vi "Detect Network Devices.vi"(4 "Remote Timeout":u32=300000 caption="Remote Timeout (300,000 ms)", 6 "Network Adapters":bool caption="Network Adapters (F)", 7 "Local Subnet Only":bool caption="Local Subnet Only (F)", 8 "Error in":errorcluster, 11 "Session in (localhost)":refnum<k21>="localhost") -> (0 "Error out":errorcluster, 1 "Devices Skipped":T1[](array[typedef]) {"Network Adapter Settings"."IP Address Request Mode" items=["Static"=1, "DHCP/Link Local"=2, "Link-Local Only"=4, "DHCP Only"=8]; "Network Adapter Settings"."Adapter Type" items=["Disabled"=1, "TCP/IP Ethernet"=2, "Deterministic"=4, "EtherCAT"=8, "TCP/IP WLAN Connect"=32, "TCP/IP WLAN Create"=64]; "Network Adapter Settings"."Adapter Mode" items=["Disabled"=1, "TCP/IP Ethernet"=2, "Deterministic"=4, "EtherCAT"=8, "TCP/IP WLAN Connect"=32, "TCP/IP WLAN Create"=64]; "Device Information"."Product ID" format="%.0x"}, 2 "Devices Found":T1[](array[typedef]) {"Network Adapter Settings"."IP Address Request Mode" items=["Static"=1, "DHCP/Link Local"=2, "Link-Local Only"=4, "DHCP Only"=8]; "Network Adapter Settings"."Adapter Type" items=["Disabled"=1, "TCP/IP Ethernet"=2, "Deterministic"=4, "EtherCAT"=8, "TCP/IP WLAN Connect"=32, "TCP/IP WLAN Create"=64]; "Network Adapter Settings"."Adapter Mode" items=["Disabled"=1, "TCP/IP Ethernet"=2, "Deterministic"=4, "EtherCAT"=8, "TCP/IP WLAN Connect"=32, "TCP/IP WLAN Create"=64]; "Device Information"."Product ID" format="%.0x"}, 3 "Session out":refnum<k21>)   [LabVIEW 2015, in "RT Management.lvlib"]
uses:
  RT Management.lvlib
  <vilib>/nisyscfg/nisyscfg.lvlib
  Controls/DeviceInformation.ctl
  Device.lvclass
  <resource>/objmgr/niflexriosae.rc
  <vilib>/nisyscfg/Filter Mode.ctl
  <vilib>/regexp/Match Regular Expression.xnode
  RT Management/Controls/DeviceClass.ctl
  RT Management/RT Management.lvclass
  Controls/NetworkAdapterSettings.ctl
  Controls/NetworkDevice.ctl
  <vilib>/nisyscfg/Close (System).vi
  <vilib>/nisyscfg/Close (Resources).vi
  <vilib>/nisyscfg/Close (Filter).vi
panel:
  in  "User Added Targets Only":bool
  in  "Reduce Discovery Timeout":bool
  in  "Device Class String":string[](array[string])
  in  "Device Class":T4
  in  "Device Class String":string
  in  "Device Class":T5
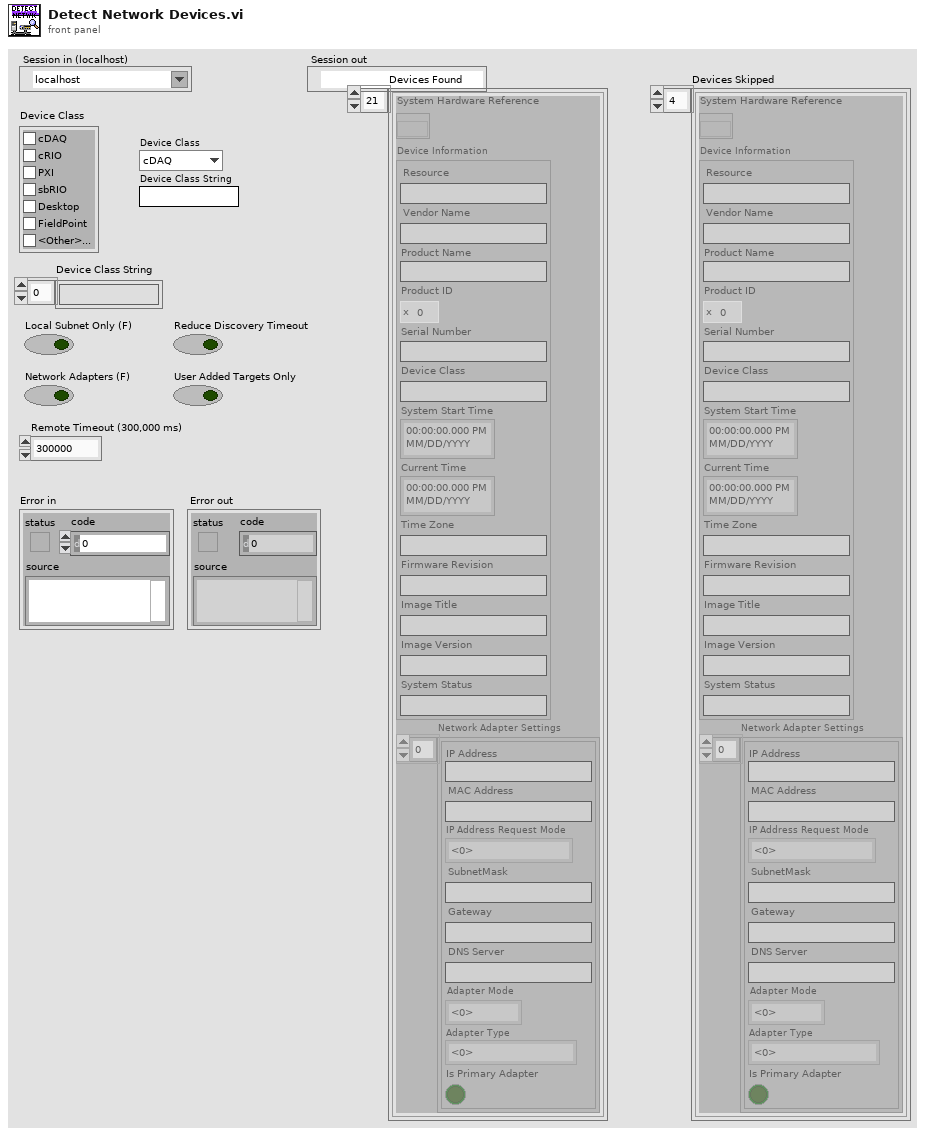
[diagram p1: front panel]
types:
  T1 = typedef "RT Management.lvlib/Device.lvclass/NetworkDevice.ctl" = cluster{"System Hardware Reference":refnum<k20>, "Device Information":T2, "Network Adapter Settings":T3[]}
  T2 = typedef "RT Management.lvlib/Device.lvclass/DeviceInformation.ctl" = cluster{"Resource":string, "Vendor Name":string, "Product Name":string, "Product ID":u32, "Serial Number":string, "Device Class":string, "System Start Time":timestamp, "Current Time":timestamp, "Time Zone":string, "Firmware Revision":string, "Image Title":string, "Image Version":string, "System Status":string}
  T3 = typedef "RT Management.lvlib/Device.lvclass/NetworkAdapterSettings.ctl" = cluster{"IP Address":string, "MAC Address":string, "IP Address Request Mode":u32, "SubnetMask":string, "Gateway":string, "DNS Server":string, "Adapter Mode":u32, "Adapter Type":u32, "Is Primary Adapter":bool}
  T4 = cluster{"cDAQ":bool, "cRIO":bool, "PXI":bool, "sbRIO":bool, "Desktop":bool, "FieldPoint":bool, "<Other>...":bool}
  T5 = typedef "RT Management.lvlib/RT Management.lvclass/DeviceClass.ctl" = enum16{"cDAQ", "cRIO", "CVS", "Ethernet RIO", "PXI", "sbRIO", "Desktop", "FieldPoint", "<Other>...", ""}
  T6 = typedef "nisyscfg.lvlib/Filter Mode.ctl" = i32
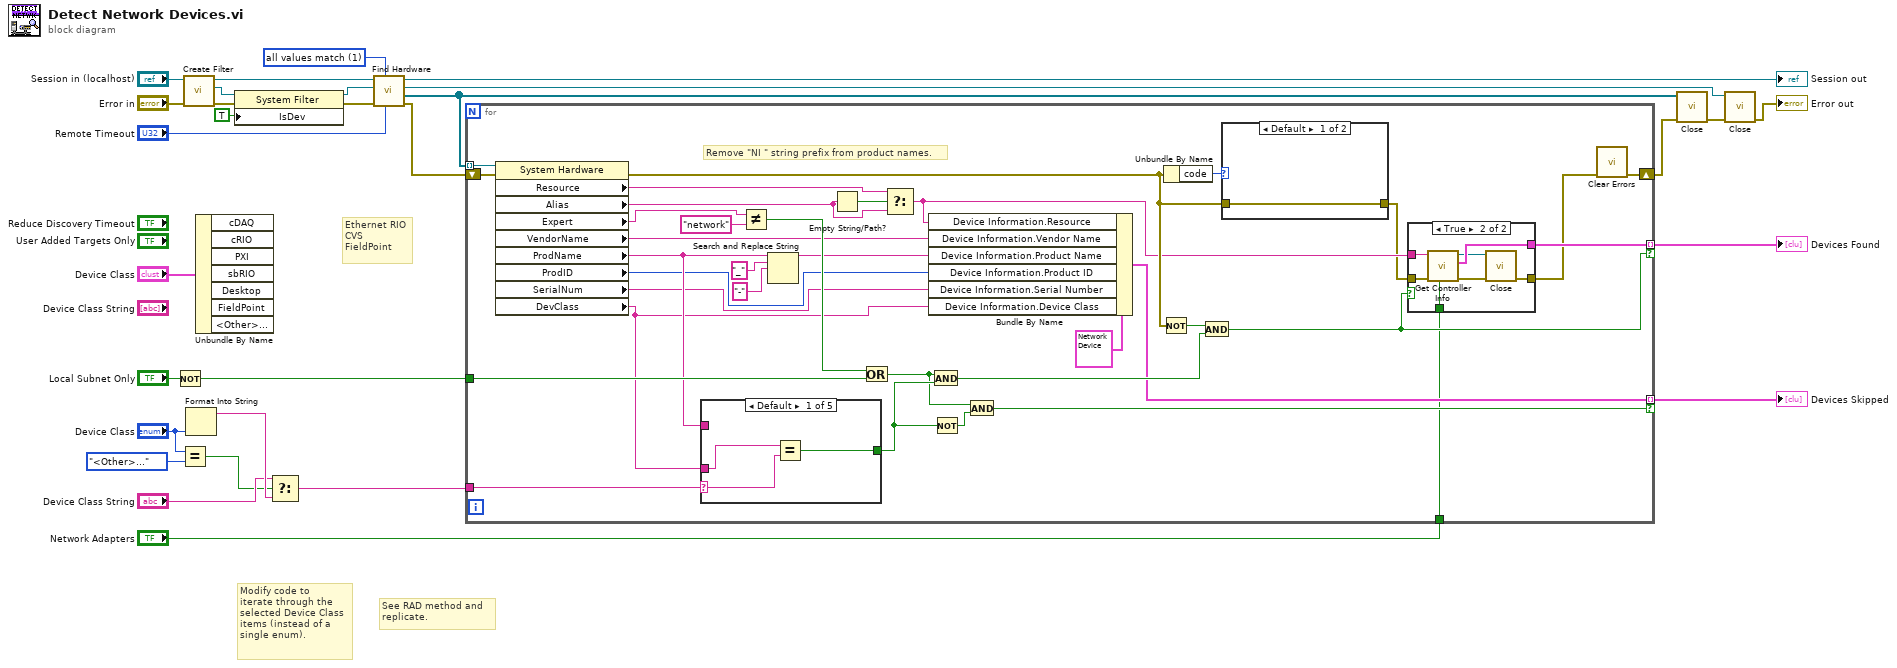
[diagram p0: block diagram]
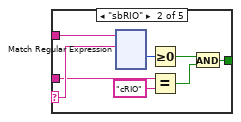
[diagram p2: hidden frame]
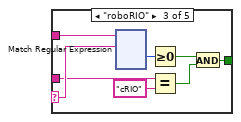
[diagram p3: hidden frame]
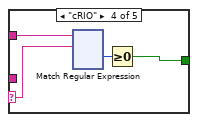
[diagram p4: hidden frame]
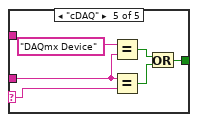
[diagram p5: hidden frame]
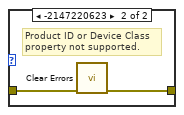
[diagram p7: hidden frame]
diagram:
  w12 = T6 1 items=["all values match"=1, "any value matches"=2, "values do not match"=3, "all properties exist"=4] ("filter mode (all values match)")
  # "Ethernet RIO\nCVS\nFieldPoint"
  # "See RAD method and\nreplicate."
  # "Modify code to\niterate through the\nselected Device Class\nitems (instead of a\nsingle enum)."
  n1 = Not(x="Local Subnet Only") -> (.not. x?=w19:bool)
  n2 = Equal?(x="Device Class", y=DeviceClass."<Other>...") -> (x = y?=w18:bool)
  n3 = call <vilib>:"Create Filter.vi"("error in (no error)"="Error in", "Session in"="Session in (localhost)") -> ("error out"=w17:errorcluster, "Filter out"=w16:refnum<k20>, "Session out"=w15:refnum<k21>)  [unwired: 7 in]
  n4 = Format Into String("Device Class") -> (resulting string=w21:string)  [unwired: 3 in, 1 out]
  n5 = Unbundle By Name("Device Class") -> ()  [unwired: 7 out]
  n6 = property class="System Filter"(reference=w16, error in=w17, "IsDev"=TRUE ("Is Chassis")) -> (reference out=w13:refnum<k20>, error out=w14:errorcluster)
  n7 = Select(t="Device Class String", s=w18, f=w21) -> (s? t:f=w29:string)
  n8 = call <vilib>:"Find Hardware.vi"("Remote Timeout (300,000 ms)"="Remote Timeout", "Filter Mode (all values match)"=w12, "error in (no error)"=w14, "Filter in"=w13, "Session in"=w15) -> ("error out"=w11:errorcluster, "Resources out"=w10:refnum<k20>[], "Filter out"=w8:refnum<k20>, "Session out"=→"Session out":refnum<k21>)  [unwired: 3 out]
  n9 = for {
    tunnel: w10 -> [w63] mode=indexing
    shift-right: [w49] -> w7
    shift-left: w11 -> [w62]
    tunnel: w19 -> [w59]
    tunnel: w29 -> [w53]
    tunnel: [w40] -> w3 mode=indexing if=w42
    tunnel: [w48] -> w4 mode=indexing if=w43
    tunnel: "Network Adapters" -> [w37]
    # "Remove \"NI \" string prefix from product names."
    n10 = property class="System Hardware"(reference=w63, error in=w62) -> (error out=w47:errorcluster, "Resource"=w57:string, "Alias"=w58:string, "Expert"=w56:string, "VendorName"=w54:string, "ProdName"=w34:string, "ProdID"=w30:u32, "SerialNum"=w31:string, "DevClass"=w32:string)  [unwired: 1 out]
    n11 = case shown="Default" w53 {
      selector: w53 -> [w67 w74 w196 w314 w432]
      tunnel: w32 -> [w66 w73 w195 _ w431]
      tunnel: w34 -> [_ w75 w197 w315 _]
      tunnel: [w65 w69 w191 w312 w433] -> w46
      frame Default {
        n12 = Equal?(x=w66, y=w67) -> (x = y?=w65:bool)
      }
      frame "sbRIO" {
        n13 = xnode "Match Regular Expression"("input string"=w75, "regular expression"=w74) -> ("offset past match"=w72:i32)  [unwired: 4 in, 4 out]
        n14 = Greater Or Equal To 0?(x=w72) -> (x >= 0?=w70:bool)
        n15 = Equal?(x=w73, y="cRIO") -> (x = y?=w71:bool)
        n16 = And(x=w70, y=w71) -> (x .and. y?=w69:bool)
      }
      frame "roboRIO" {
        n17 = xnode "Match Regular Expression"("input string"=w197, "regular expression"=w196) -> ("offset past match"=w194:i32)  [unwired: 4 in, 4 out]
        n18 = Greater Or Equal To 0?(x=w194) -> (x >= 0?=w192:bool)
        n19 = Equal?(x=w195, y="cRIO") -> (x = y?=w193:bool)
        n20 = And(x=w192, y=w193) -> (x .and. y?=w191:bool)
      }
      frame "cRIO" {
        n21 = xnode "Match Regular Expression"("input string"=w315, "regular expression"=w314) -> ("offset past match"=w313:i32)  [unwired: 4 in, 4 out]
        n22 = Greater Or Equal To 0?(x=w313) -> (x >= 0?=w312:bool)
      }
      frame "cDAQ" {
        n23 = Equal?(x="DAQmx Device", y=w431) -> (x = y?=w435:bool)
        n24 = Equal?(x=w431, y=w432) -> (x = y?=w434:bool)
        n25 = Or(x=w435, y=w434) -> (x .or. y?=w433:bool)
      }
    }
    n26 = Not Equal?(x=w56, y="network") -> (x != y?=w60:bool)
    n27 = Search and Replace String(input string=w34, search string="_", replace string="-" ("replace string (\"\")")) -> (result string=w33:string)  [unwired: 5 in, 3 out]
    n28 = Empty String/Path?(string/path=w58) -> (empty?=w64:bool)
    n29 = Or(x=w60, y=w59) -> (x .or. y?=w44:bool)
    n30 = Select(t=w57, s=w64, f=w58) -> (s? t:f=w41:string)
    n31 = Bundle By Name(cluster=T1 {"System Hardware Reference"=refnum, "Device Information"={"Resource"="", "Vendor Name"="", "Product Name"="", "Product ID"=0, "Serial Number"="", "Device Class"="", "System Start Time"=timestamp(0 s since 1904-01-01), "Current Time"=timestamp(0 s since 1904-01-01), "Time Zone"="", "Firmware Revision"="", "Image Title"="", "Image Version"="", "System Status"=""}, "Network Adapter Settings"=[]} ("Device Information"), "Device Information.Resource"=w41, "Device Information.Vendor Name"=w54, "Device Information.Product Name"=w33, "Device Information.Product ID"=w30, "Device Information.Serial Number"=w31, "Device Information.Device Class"=w32) -> (w48:T1)
    n32 = And(x=w44, y=w46) -> (x .and. y?=w52:bool)
    n33 = Not(x=w46) -> (.not. x?=w45:bool)
    n34 = And(x=w44, y=w45) -> (x .and. y?=w43:bool)
    n35 = Not(x=w47) -> (.not. x?=w51:bool)
    n36 = Unbundle By Name(w47) -> ("code"=w50:i32)
    n37 = And(x=w51, y=w52) -> (x .and. y?=w42:bool)
    n38 = case shown="Default" w50 {
      tunnel: w47 -> [w444 w446]
      tunnel: [w444 w445] -> w39
      frame Default {
      }
      frame -2147220623 {
        # "Product ID or Device Class\nproperty not supported."
        n39 = call <vilib>:"Clear Errors.vi"("error in (no error)"=w446) -> ("error out"=w445:errorcluster)  [unwired: 5 in, 1 out]
      }
    }
    n40 = case shown="True" w42 {
      tunnel: w41 -> [_ w443]
      tunnel: [_ w442] -> w40
      tunnel: w39 -> [w436 w439]
      tunnel: [w436 w438] -> w38
      tunnel: w37 -> [_ w437]
      frame False {
      }
      frame True {
        n41 = call "Get Controller Info.vi"("Network Adapters"=w437, "error in"=w439, "Session in"=w443) -> ("error out"=w441:errorcluster, "Network Device"=w442:T1, "Session out"=w440:refnum<k21>)  [unwired: 6 in]
        n42 = call-poly <vilib>:"Close.vi"("error in (no error)"=w441, "Session in"=w440) -> ("error out"=w438:errorcluster)  [unwired: 9 in]
      }
    }
    n43 = call <vilib>:"Clear Errors.vi"("error in (no error)"=w38) -> ("error out"=w49:errorcluster)  [unwired: 5 in, 1 out]
  }
  "Devices Found" <- w3
  "Devices Skipped" <- w4
  n44 = call-poly <vilib>:"Close.vi"("error in (no error)"=w7, "Resources in"=w10) -> ("error out"=w6:errorcluster)  [unwired: 9 in]
  n45 = call-poly <vilib>:"Close.vi"("error in (no error)"=w6, "Filter in"=w8) -> ("error out"=→"Error out":errorcluster)  [unwired: 9 in]
